vi "NI PXIe-411x PS Ch Page.vi"(8 "error in (no error)":errorcluster, 11 "Node Ptr":T2 format="%.0x") -> (0 "error out":errorcluster)   [LabVIEW 2023, in "NI PXIe-411x PS Custom Device.lvlib"]
uses:
  NI PXIe-411x PS Custom Device.lvlib
  <vilib>/NI VeriStand/Custom Device API/Custom Device Item Ref.ctl
  411x_Channel #.ctl
  411x_Global.vi
  <vilib>/NI VeriStand/Custom Device API/Get Item Property (Boolean).vi
  <vilib>/NI VeriStand/Custom Device API/Get Item Property (U16).vi
  <vilib>/NI VeriStand/Custom Device API/Get Item Property (Double).vi
  <vilib>/NI VeriStand/Custom Device API/Get Item Property (I32).vi
  <vilib>/NI VeriStand/Custom Device API/Set Item Property (I32).vi
  <vilib>/NI VeriStand/Custom Device API/Set Item Property (U16).vi
  <vilib>/NI VeriStand/Custom Device API/Set Item Property (Double).vi
  <vilib>/NI VeriStand/Custom Device API/Custom Device API.lvlib
panel:
  in  "Sense":i32(ring) items=["Local"=1008, "Remote"=1009]
  in  "Channel #":T1
  in  "Voltage Limit":dbl caption="Range (0-6V)" format="%.4f"
  in  "Initial Current Value":dbl caption="Range (0.01 -1A)" format="%.4f"
  in  "Current Limit":dbl caption="Range (0.01-1A)" format="%.4f"
  in  "IO Type":enum16{"Voltage Output", "Current Output"}(ring)
  in  "Voltage Level":dbl caption="Range (0-6V)" format="%_4f"
  in  "Name":string
  in  "Header":cluster{"Section Name":string}={"Section Name"="PXI-4112  Settings"}
  in  "Description":string
  in  "Delete":bool
  # "Voltage  IO Settings"
  # "Current IO Settings"
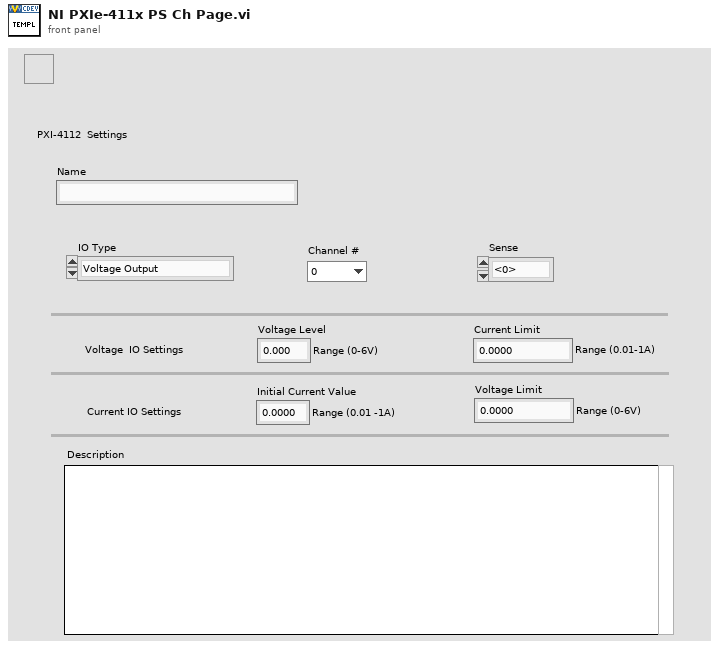
[diagram p1: front panel]
types:
  T1 = typedef "NI PXIe-411x PS Custom Device.lvlib/411x_Channel #.ctl" = enum16{"0", "1"}
  T2 = typedef "Custom Device API.lvlib/Custom Device Item Ref.ctl" = u64
  T3 = enum8{"Enabled", "Disabled", "Disabled and Grayed Out"}
  T4 = cluster{"V_min":dbl, "V_max":dbl, "I_min":dbl, "I_max":dbl}
  T5 = typedef "Custom Device API.lvlib/Custom Device Item Info.ctl" = cluster{"Name":string, "Is Channel":bool, "GUID":string, "Is Waveform":bool}
  T6 = typedef "Custom Device API.lvlib/Custom Device Commands.ctl" = enum16{"Default", "Item renamed", "Shutdown", "Dynamic button pressed"}
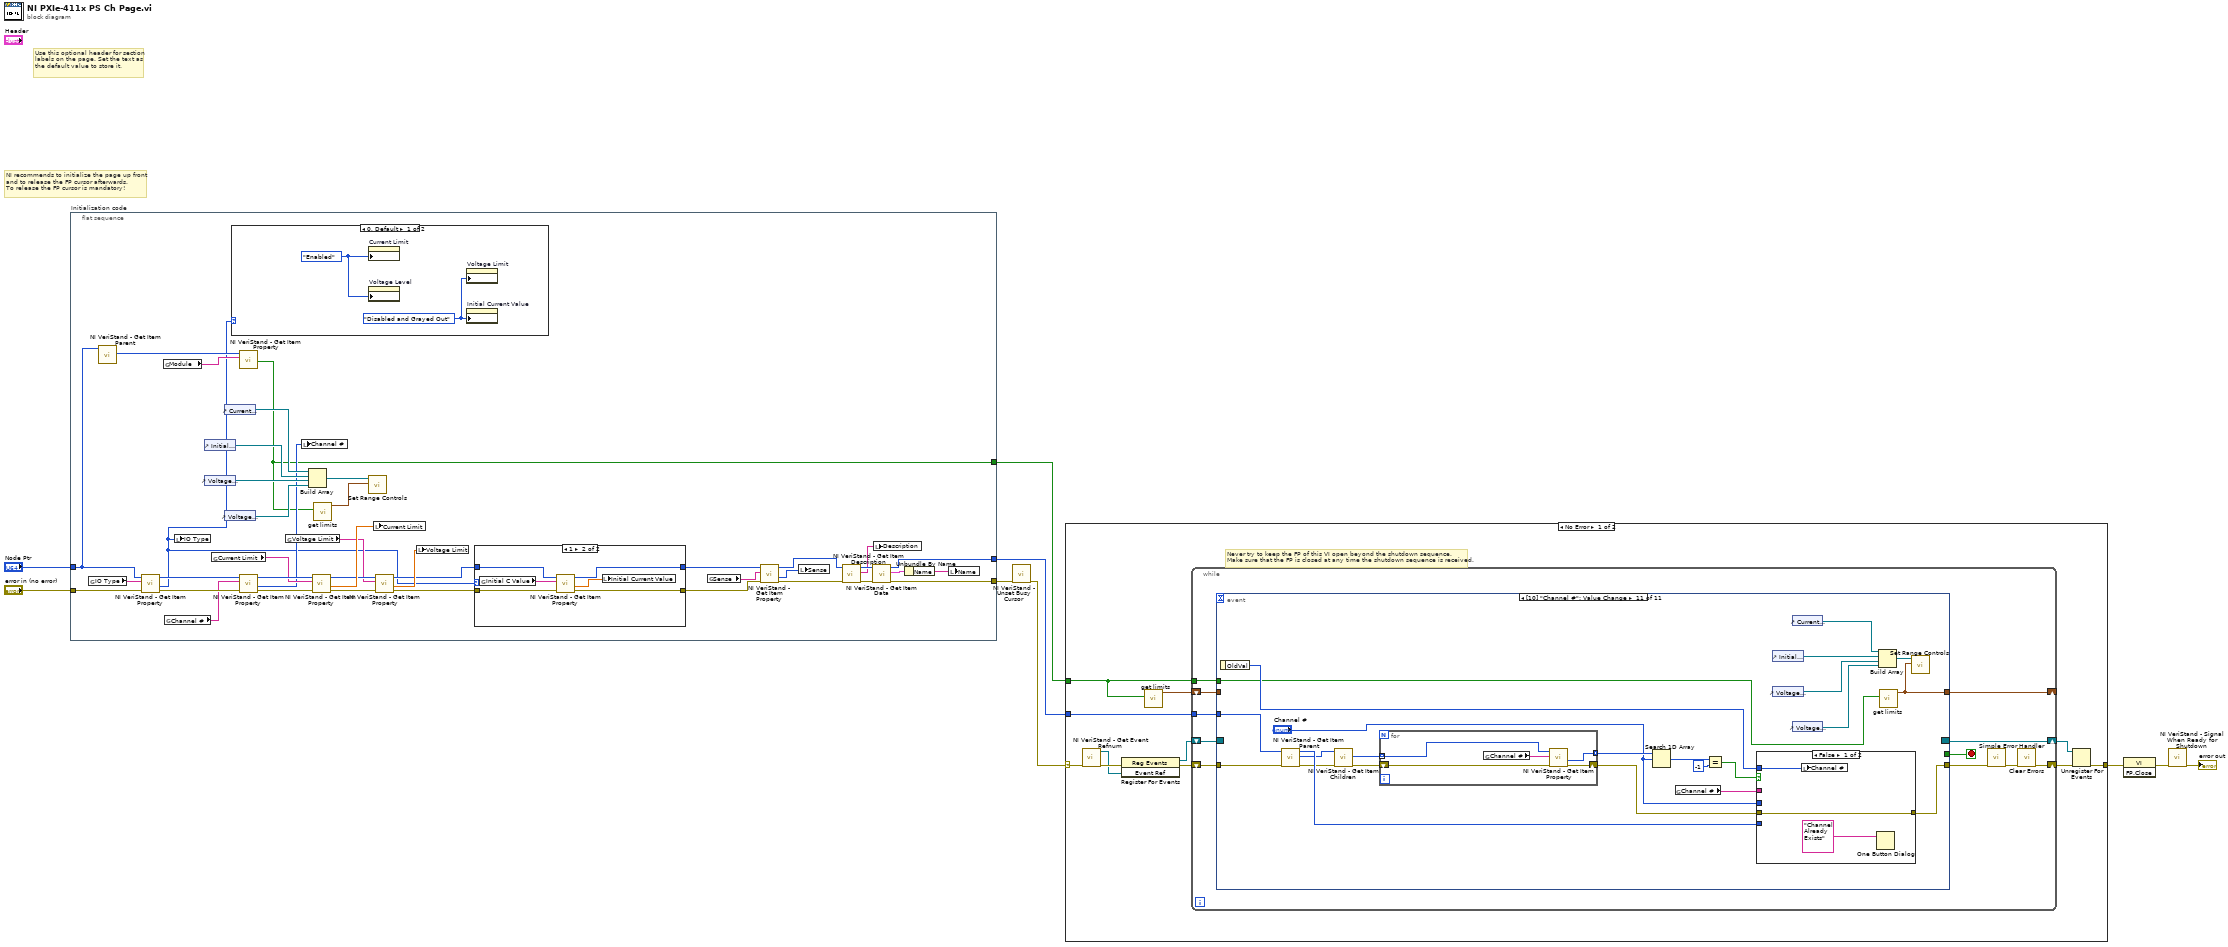
[diagram p0: block diagram]
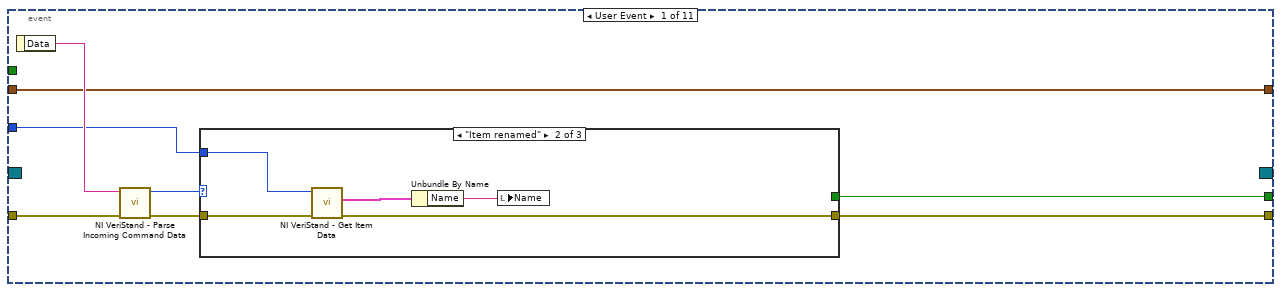
[diagram p2: hidden frame]
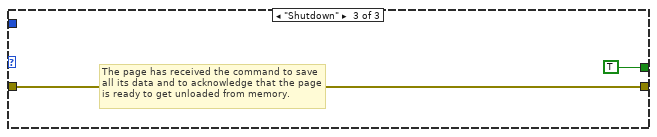
[diagram p4: hidden frame]
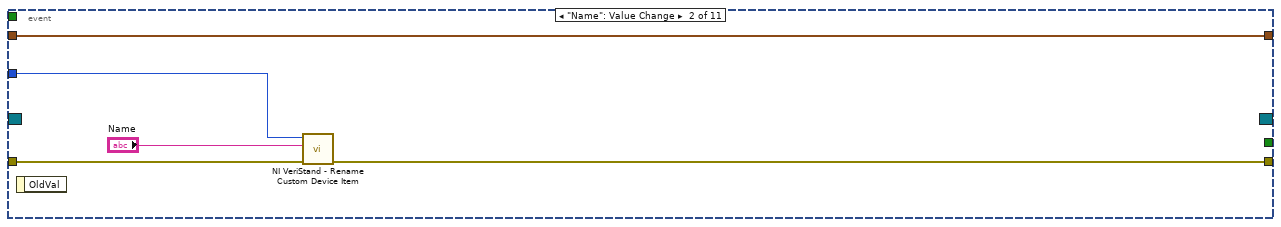
[diagram p5: hidden frame]
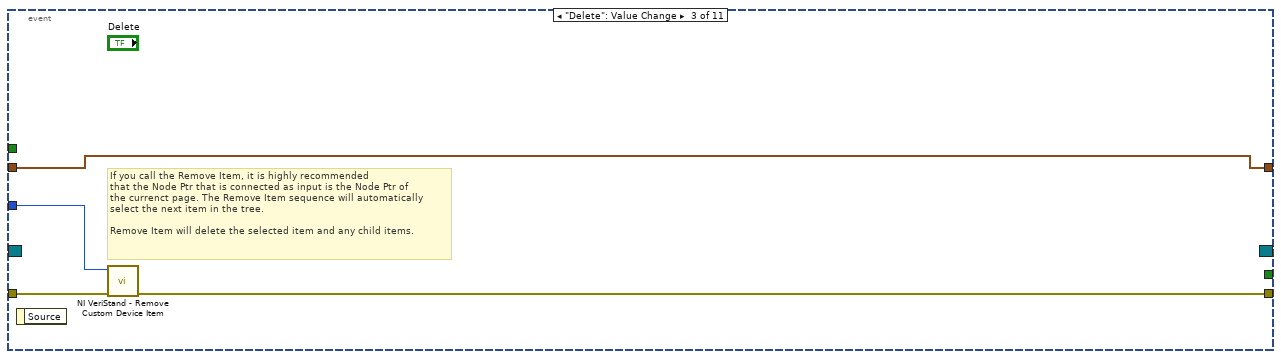
[diagram p6: hidden frame]
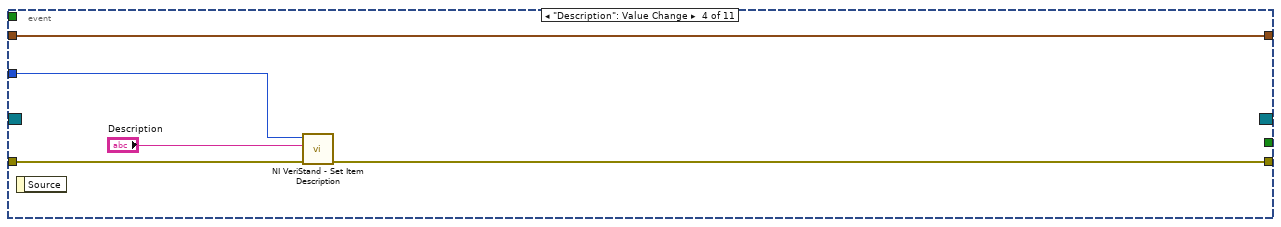
[diagram p7: hidden frame]
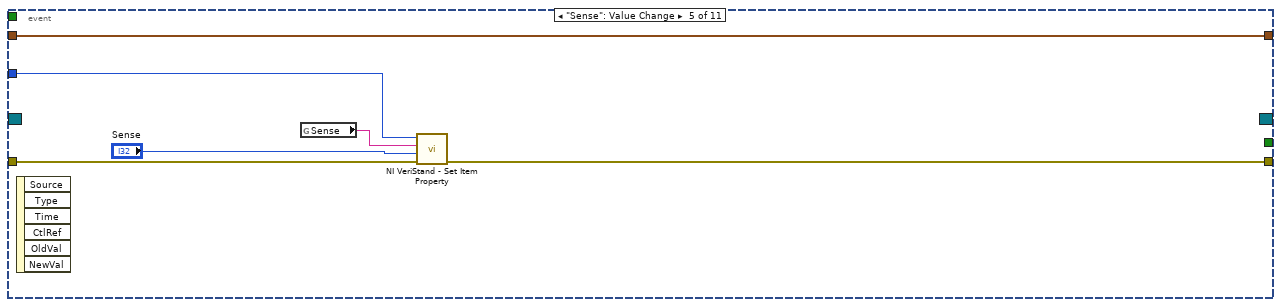
[diagram p8: hidden frame]
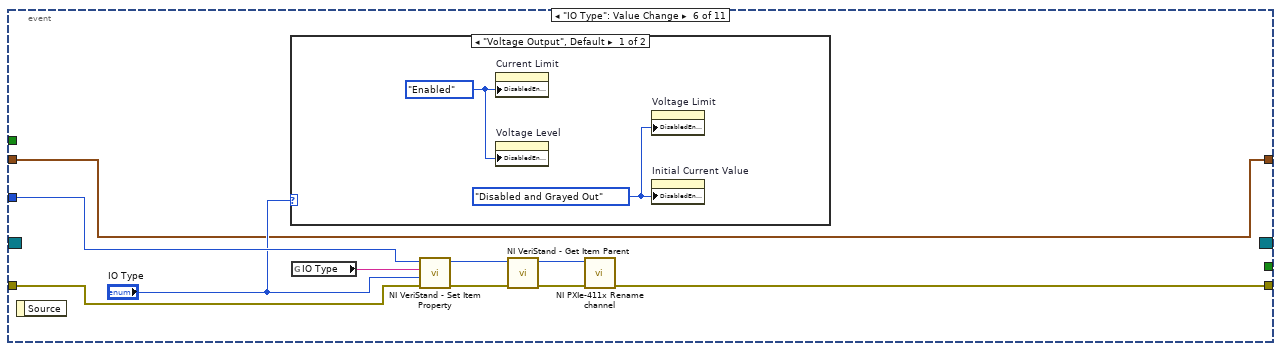
[diagram p9: hidden frame]
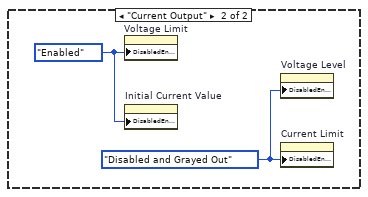
[diagram p10: hidden frame]
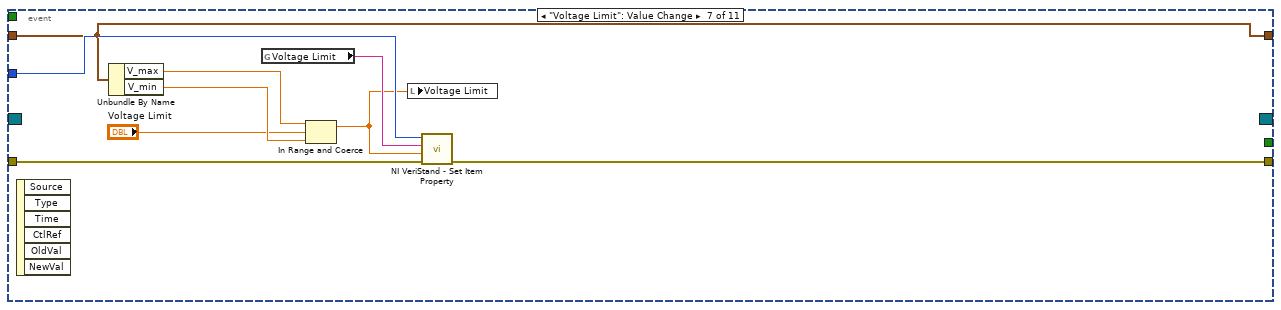
[diagram p11: hidden frame]
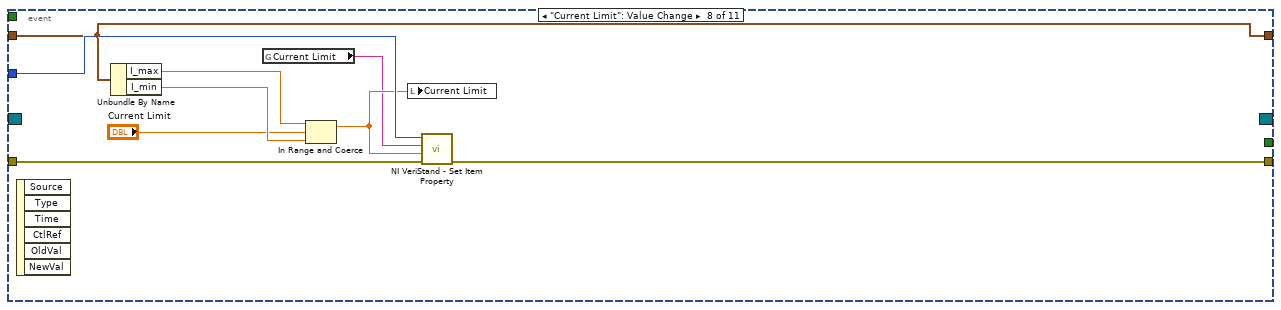
[diagram p12: hidden frame]
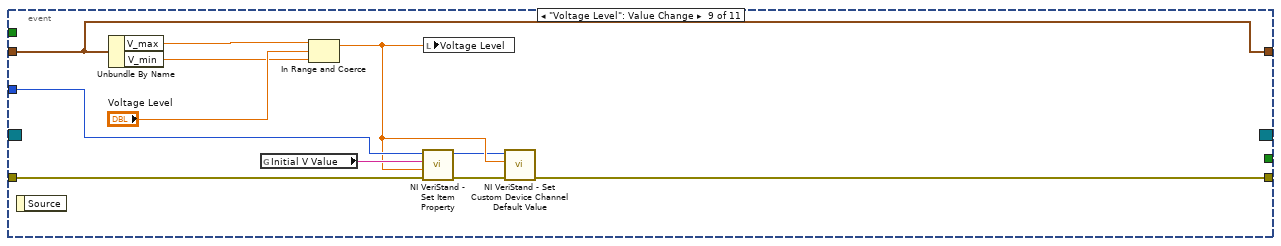
[diagram p13: hidden frame]
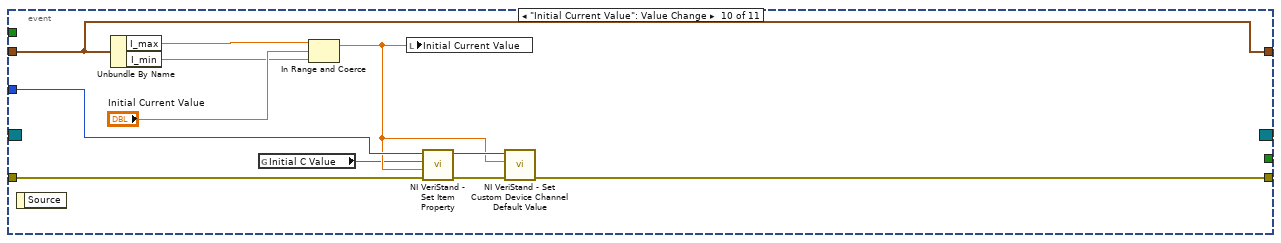
[diagram p14: hidden frame]
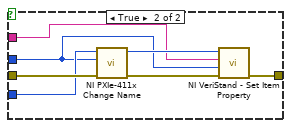
[diagram p15: hidden frame]
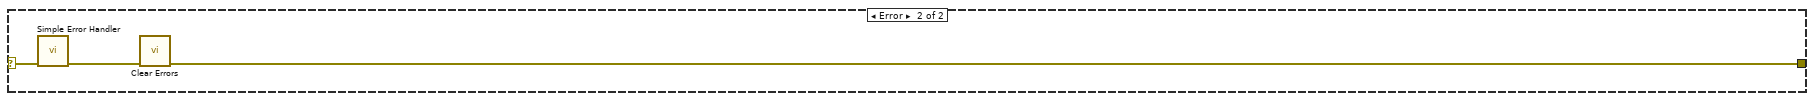
[diagram p16: hidden frame]
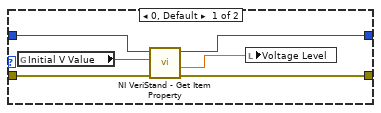
[diagram p17: hidden frame]
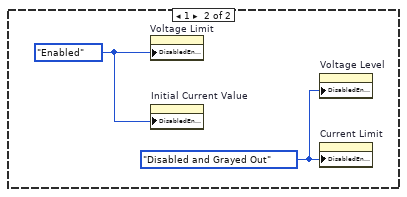
[diagram p18: hidden frame]
diagram:
  # "Use this optional header for section labels on the page. Set the text as the default value to store it."
  # "NI recommends to initialize the page up front\nand to release the FP cursor afterwards.\nTo release the FP cursor is mandatory!"
  n1 = flat-sequence "Initialization code" {
    tunnel: "error in (no error)" -> [w42]
    tunnel: "Node Ptr" -> [w21]
    tunnel: [w44] -> w5
    tunnel: [w49] -> w3
    tunnel: [w11] -> w1
    frame #0 {
      n2 = global read "411x_Global.vi" "IO Type"() -> (w41:string)
      n3 = call <vilib>:"NI VeriStand - Get Item Parent.vi"("Item Ref in"=w21) -> ("Parent Ref"=w19:T2)  [unwired: 7 in, 3 out]
      n4 = call-poly <vilib>:"NI VeriStand - Get Item Property.vi"("error in (no error)"=w42, "Property Name"=w41, "Item Ref in"=w21) -> ("error out"=w40:errorcluster, "Value"=w10:u16, "Item Ref out"=w39:T2)  [unwired: 5 in, 1 out]
      n5 = global read "411x_Global.vi" "Module"() -> (w20:string)
      n6 = global read "411x_Global.vi" "Channel #"() -> (w38:string)
      n7 = local write "IO Type"(w10) -> ()
      n8 = control-ref of="Initial Current Value"() -> (w15:refnum<vi>)
      n9 = control-ref of="Voltage Level"() -> (w16:refnum<vi>)
      n10 = global read "411x_Global.vi" "Current Limit"() -> (w35:string)
      n11 = control-ref of="Current Limit"() -> (w14:refnum<vi>)
      n12 = control-ref of="Voltage Limit"() -> (w17:refnum<vi>)
      n13 = case shown="0, Default" w10 {
        frame 0, Default {
          w62 = T3."Enabled" ("Disabled")
          w63 = T3."Disabled and Grayed Out" ("Disabled")
          n14 = property on="Current Limit" class="DigNum (strict)"("DisabledEnum"=w62) -> ()  [unwired: 2 in, 2 out]
          n15 = property on="Voltage Level" class="DigNum (strict)"("DisabledEnum"=w62) -> ()  [unwired: 2 in, 2 out]
          n16 = property on="Voltage Limit" class="DigNum (strict)"("DisabledEnum"=w63) -> ()  [unwired: 2 in, 2 out]
          n17 = property on="Initial Current Value" class="DigNum (strict)"("DisabledEnum"=w63) -> ()  [unwired: 2 in, 2 out]
        }
        frame 1 {
          w64 = T3."Enabled" ("Disabled")
          w65 = T3."Disabled and Grayed Out" ("Disabled")
          n18 = property on="Voltage Limit" class="DigNum (strict)"("DisabledEnum"=w64) -> ()  [unwired: 2 in, 2 out]
          n19 = property on="Initial Current Value" class="DigNum (strict)"("DisabledEnum"=w64) -> ()  [unwired: 2 in, 2 out]
          n20 = property on="Voltage Level" class="DigNum (strict)"("DisabledEnum"=w65) -> ()  [unwired: 2 in, 2 out]
          n21 = property on="Current Limit" class="DigNum (strict)"("DisabledEnum"=w65) -> ()  [unwired: 2 in, 2 out]
        }
      }
      n22 = call-poly <vilib>:"NI VeriStand - Get Item Property.vi"("Property Name"=w20, "Item Ref in"=w19) -> ("Value"=w11:bool)  [unwired: 6 in, 3 out]
      n23 = call-poly <vilib>:"NI VeriStand - Get Item Property.vi"("error in (no error)"=w40, "Property Name"=w38, "Item Ref in"=w39) -> ("error out"=w36:errorcluster, "Value"=w12:u16, "Item Ref out"=w37:T2)  [unwired: 5 in, 1 out]
      n24 = global read "411x_Global.vi" "Voltage Limit"() -> (w31:string)
      n25 = local write "Channel #"(w12) -> ()
      n26 = Build Array(w14, w15, w16, w17) -> (w18:refnum<vi>[])
      n27 = call-poly <vilib>:"NI VeriStand - Get Item Property.vi"("error in (no error)"=w36, "Property Name"=w35, "Item Ref in"=w37) -> ("error out"=w33:errorcluster, "Value"=w34:dbl, "Item Ref out"=w32:T2)  [unwired: 5 in, 1 out]
      n28 = call "get limits.vi"("4112?"=w11) -> ("output cluster"=w13:T4)  [unwired: 10 in]
      n29 = call "Set Range Controls.vi"("Ranges"=w13, "Reference Array"=w18) -> ()  [unwired: 10 in]
      n30 = local write "Current Limit"(w34) -> ()
      n31 = call-poly <vilib>:"NI VeriStand - Get Item Property.vi"("error in (no error)"=w33, "Property Name"=w31, "Item Ref in"=w32) -> ("error out"=w28:errorcluster, "Value"=w30:dbl, "Item Ref out"=w29:T2)  [unwired: 5 in, 1 out]
      n32 = local write "Voltage Limit"(w30) -> ()
      n33 = case shown="1" w10 {
        tunnel: w29 -> [w55 w61]
        tunnel: w28 -> [w54 w60]
        tunnel: [w53 w59] -> w26
        tunnel: [w52 w58] -> w25
        frame 0, Default {
          n34 = global read "411x_Global.vi" "Initial V Value"() -> (w51:string)
          n35 = call-poly <vilib>:"NI VeriStand - Get Item Property.vi"("error in (no error)"=w54, "Property Name"=w51, "Item Ref in"=w55) -> ("error out"=w53:errorcluster, "Value"=w50:dbl, "Item Ref out"=w52:T2)  [unwired: 5 in, 1 out]
          n36 = local write "Voltage Level"(w50) -> ()
        }
        frame 1 {
          n37 = global read "411x_Global.vi" "Initial C Value"() -> (w57:string)
          n38 = call-poly <vilib>:"NI VeriStand - Get Item Property.vi"("error in (no error)"=w60, "Property Name"=w57, "Item Ref in"=w61) -> ("error out"=w59:errorcluster, "Value"=w56:dbl, "Item Ref out"=w58:T2)  [unwired: 5 in, 1 out]
          n39 = local write "Initial Current Value"(w56) -> ()
        }
      }
      n40 = global read "411x_Global.vi" "Sense"() -> (w24:string)
      n41 = call-poly <vilib>:"NI VeriStand - Get Item Property.vi"("error in (no error)"=w26, "Property Name"=w24, "Item Ref in"=w25) -> ("error out"=w22:errorcluster, "Value"=w27:i32, "Item Ref out"=w23:T2)  [unwired: 5 in, 1 out]
      n42 = local write "Sense"(w27) -> ()
      n43 = call <vilib>:"NI VeriStand - Get Item Description.vi"("error in (no error)"=w22, "Item Ref in"=w23) -> ("error out"=w46:errorcluster, "Description"=w47:string, "Item Ref out"=w48:T2)  [unwired: 7 out]
      n44 = call <vilib>:"NI VeriStand - Get Item Data.vi"("error in (no error)"=w46, "Item Ref in"=w48) -> ("error out"=w44:errorcluster, "Item Info"=w45:T5, "Item Ref out"=w49:T2)  [unwired: 7 out]
      n45 = local write "Description"(w47) -> ()
      n46 = Unbundle By Name(w45) -> ("Name"=w43:string)
      n47 = local write "Name"(w43) -> ()
    }
  }
  n48 = call <vilib>:"NI VeriStand - Unset Busy Cursor.vi"("error in (no error)"=w5) -> ("error out"=w4:errorcluster)  [unwired: 10 out]
  n49 = case shown="No Error" w4 {
    selector: w4 -> [w68 w218]
    tunnel: [w73 w216] -> w9
    tunnel: w3 -> [w69 _]
    tunnel: w1 -> [w66 _]
    frame No Error {
      # "Never try to keep the FP of this VI open beyond the shutdown sequence.\nMake sure that the FP is closed at any time the shutdown sequence is received."
      n50 = call <vilib>:"NI VeriStand - Get Event Refnum.vi"("error in (no error)"=w68) -> ("error out"=w76:errorcluster, "Event Ref"=w72:refnum<user-event>)  [unwired: 9 out]
      n51 = register-events(error in=w76, w72) -> (reference out=w70:refnum<event-registration>, error out=w71:errorcluster)  [unwired: 1 in]
      n52 = call "get limits.vi"("4112?"=w66) -> ("output cluster"=w67:T4)  [unwired: 10 in]
      n53 = while {
        tunnel: w69 -> [w83]
        shift-right: [w80] -> w74
        shift-left: w71 -> [w86]
        shift-right: [w87] -> w75
        shift-left: w70 -> [w85]
        shift-right: [w79] -> _
        shift-left: w67 -> [w78]
        tunnel: w66 -> [w77]
        stop <- w84 stop-if-true
        n54 = event shown="[10] \"Channel #\": Value Change" {
          selector: w85 -> [_ _ _ _ _ _ _ _ _ _ _]
          dyn-events: [_ _ _ _ _ _ _ _ _ _ _] -> w87
          timeout: _ -> [_ _ _ _ _ _ _ _ _ _ _]
          tunnel: w86 -> [w95 w108 w112 w116 w123 w132 w145 w154 w165 w176 w187]
          tunnel: [w91 _ _ _ _ _ _ _ _ _ _] -> w84
          tunnel: [w90 w107 w111 w115 w122 w126 w144 w153 w162 w174 w186] -> w82
          tunnel: w83 -> [w89 w106 w110 w117 w121 w133 w146 w155 w166 w177 w188]
          tunnel: [w88 w104 w109 w113 w120 w124 w142 w150 w158 w171 w178] -> w79
          tunnel: w78 -> [w88 w104 w109 w113 w120 w124 w142 w150 w158 w171 _]
          tunnel: w77 -> [_ _ _ _ _ _ _ _ _ _ w184]
          event User Event {
            n55 = event-data() -> ("Data"=w94:string)  [unwired: 1 out]
            n56 = call <vilib>:"NI VeriStand - Parse Incoming Command Data.vi"("error in (no error)"=w95, "Incoming data"=w94) -> ("error out"=w93:errorcluster, "Action"=w92:T6)  [unwired: 8 out]
            n57 = case shown="\"Item renamed\"" w92 {
              tunnel: w93 -> [w96 w101 w102]
              tunnel: [_ _ TRUE] -> w91
              tunnel: [w96 w98 w102] -> w90
              tunnel: w89 -> [_ w100 _]
              frame "Default", Default {
              }
              frame "Item renamed" {
                n58 = call <vilib>:"NI VeriStand - Get Item Data.vi"("error in (no error)"=w101, "Item Ref in"=w100) -> ("error out"=w98:errorcluster, "Item Info"=w99:T5)  [unwired: 8 out]
                n59 = Unbundle By Name(w99) -> ("Name"=w97:string)
                n60 = local write "Name"(w97) -> ()
              }
              frame "Shutdown" {
                # "The page has received the command to save all its data and to acknowledge that the page is ready to get unloaded from memory."
              }
            }
          }
          event "Name": Value Change {
            n61 = event-data() -> ()  [unwired: 2 out]
            n62 = call <vilib>:"NI VeriStand - Rename Custom Device Item.vi"("error in (no error)"=w108, "New Name"="Name", "Item Ref in"=w106) -> ("error out"=w107:errorcluster)  [unwired: 1 in, 7 out]
          }
          event "Delete": Value Change {
            # "If you call the Remove Item, it is highly recommended\nthat the Node Ptr that is connected as input is the Node Ptr of\nthe currenct page. The Remove Item sequence will automatically\nselect the next item in the tree.\n\nRemove Item will delete the selected item and any child items."
            n63 = event-data() -> ()  [unwired: 2 out]
            n64 = call <vilib>:"NI VeriStand - Remove Custom Device Item.vi"("error in (no error)"=w112, "Item Ref in"=w110) -> ("error out"=w111:errorcluster)  [unwired: 1 in, 8 out]
          }
          event "Description": Value Change {
            n65 = event-data() -> ()  [unwired: 2 out]
            n66 = call <vilib>:"NI VeriStand - Set Item Description.vi"("error in (no error)"=w116, "Description"="Description", "Item Ref in"=w117) -> ("error out"=w115:errorcluster)  [unwired: 8 out]
          }
          event "Sense": Value Change {
            n67 = event-data() -> ()  [unwired: 7 out]
            n68 = global read "411x_Global.vi" "Sense"() -> (w119:string)
            n69 = call-poly <vilib>:"NI VeriStand - Set Item Property.vi"("error in (no error)"=w123, "Value"="Sense", "Property Name"=w119, "Item Ref in"=w121) -> ("error out"=w122:errorcluster)  [unwired: 5 in, 2 out]
          }
          event "IO Type": Value Change {
            n70 = event-data() -> ()  [unwired: 2 out]
            n71 = case shown="\"Voltage Output\", Default" "IO Type" {
              frame "Voltage Output", Default {
                w134 = T3."Enabled" ("Disabled")
                w135 = T3."Disabled and Grayed Out" ("Disabled")
                n72 = property on="Current Limit" class="DigNum (strict)"("DisabledEnum"=w134) -> ()  [unwired: 2 in, 2 out]
                n73 = property on="Voltage Level" class="DigNum (strict)"("DisabledEnum"=w134) -> ()  [unwired: 2 in, 2 out]
                n74 = property on="Voltage Limit" class="DigNum (strict)"("DisabledEnum"=w135) -> ()  [unwired: 2 in, 2 out]
                n75 = property on="Initial Current Value" class="DigNum (strict)"("DisabledEnum"=w135) -> ()  [unwired: 2 in, 2 out]
              }
              frame "Current Output" {
                w136 = T3."Enabled" ("Disabled")
                w137 = T3."Disabled and Grayed Out" ("Disabled")
                n76 = property on="Voltage Limit" class="DigNum (strict)"("DisabledEnum"=w136) -> ()  [unwired: 2 in, 2 out]
                n77 = property on="Initial Current Value" class="DigNum (strict)"("DisabledEnum"=w136) -> ()  [unwired: 2 in, 2 out]
                n78 = property on="Voltage Level" class="DigNum (strict)"("DisabledEnum"=w137) -> ()  [unwired: 2 in, 2 out]
                n79 = property on="Current Limit" class="DigNum (strict)"("DisabledEnum"=w137) -> ()  [unwired: 2 in, 2 out]
              }
            }
            n80 = global read "411x_Global.vi" "IO Type"() -> (w131:string)
            n81 = call-poly <vilib>:"NI VeriStand - Set Item Property.vi"("error in (no error)"=w132, "Value"="IO Type", "Property Name"=w131, "Item Ref in"=w133) -> ("error out"=w129:errorcluster, "Item Ref out"=w127:T2)  [unwired: 5 in, 1 out]
            n82 = call <vilib>:"NI VeriStand - Get Item Parent.vi"("error in (no error)"=w129, "Item Ref in"=w127) -> ("error out"=w125:errorcluster, "Item Ref out"=w128:T2)  [unwired: 6 in, 2 out]
            n83 = call "NI PXIe-411x Rename channel.vi"("error in (no error)"=w125, "Node Ptr"=w128) -> ("error out"=w126:errorcluster)  [unwired: 8 in, 1 out]
          }
          event "Voltage Limit": Value Change {
            n84 = event-data() -> ()  [unwired: 7 out]
            n85 = Unbundle By Name(w142) -> ("V_max"=w141:dbl, "V_min"=w140:dbl)
            n86 = global read "411x_Global.vi" "Voltage Limit"() -> (w143:string)
            n87 = In Range and Coerce(upper limit=w141, x="Voltage Limit", lower limit=w140) -> (coerced(x)=w138:dbl)  [unwired: 1 out]
            n88 = local write "Voltage Limit"(w138) -> ()
            n89 = call-poly <vilib>:"NI VeriStand - Set Item Property.vi"("error in (no error)"=w145, "Value"=w138, "Property Name"=w143, "Item Ref in"=w146) -> ("error out"=w144:errorcluster)  [unwired: 5 in, 2 out]
          }
          event "Current Limit": Value Change {
            n90 = event-data() -> ()  [unwired: 7 out]
            n91 = Unbundle By Name(w150) -> ("I_max"=w152:dbl, "I_min"=w151:dbl)
            n92 = global read "411x_Global.vi" "Current Limit"() -> (w147:string)
            n93 = In Range and Coerce(upper limit=w152, x="Current Limit", lower limit=w151) -> (coerced(x)=w148:dbl)  [unwired: 1 out]
            n94 = local write "Current Limit"(w148) -> ()
            n95 = call-poly <vilib>:"NI VeriStand - Set Item Property.vi"("error in (no error)"=w154, "Value"=w148, "Property Name"=w147, "Item Ref in"=w155) -> ("error out"=w153:errorcluster)  [unwired: 5 in, 2 out]
          }
          event "Voltage Level": Value Change {
            n96 = event-data() -> ()  [unwired: 2 out]
            n97 = Unbundle By Name(w158) -> ("V_max"=w157:dbl, "V_min"=w156:dbl)
            n98 = global read "411x_Global.vi" "Initial V Value"() -> (w164:string)
            n99 = In Range and Coerce(upper limit=w157, x="Voltage Level", lower limit=w156) -> (coerced(x)=w161:dbl)  [unwired: 1 out]
            n100 = call-poly <vilib>:"NI VeriStand - Set Item Property.vi"("error in (no error)"=w165, "Value"=w161, "Property Name"=w164, "Item Ref in"=w166) -> ("error out"=w163:errorcluster, "Item Ref out"=w160:T2)  [unwired: 5 in, 1 out]
            n101 = local write "Voltage Level"(w161) -> ()
            n102 = call <vilib>:"NI VeriStand - Set Custom Device Channel Default Value.vi"("error in (no error)"=w163, "Default Value"=w161, "Channel Ref in"=w160) -> ("error out"=w162:errorcluster)  [unwired: 7 in, 1 out]
          }
          event "Initial Current Value": Value Change {
            n103 = event-data() -> ()  [unwired: 2 out]
            n104 = Unbundle By Name(w171) -> ("I_max"=w170:dbl, "I_min"=w169:dbl)
            n105 = global read "411x_Global.vi" "Initial C Value"() -> (w167:string)
            n106 = In Range and Coerce(upper limit=w170, x="Initial Current Value", lower limit=w169) -> (coerced(x)=w168:dbl)  [unwired: 1 out]
            n107 = local write "Initial Current Value"(w168) -> ()
            n108 = call-poly <vilib>:"NI VeriStand - Set Item Property.vi"("error in (no error)"=w176, "Value"=w168, "Property Name"=w167, "Item Ref in"=w177) -> ("error out"=w175:errorcluster, "Item Ref out"=w173:T2)  [unwired: 5 in, 1 out]
            n109 = call <vilib>:"NI VeriStand - Set Custom Device Channel Default Value.vi"("error in (no error)"=w175, "Default Value"=w168, "Channel Ref in"=w173) -> ("error out"=w174:errorcluster)  [unwired: 7 in, 1 out]
          }
          event Value Change {
            n110 = event-data() -> ("OldVal"=w190:T1)  [unwired: 1 out]
            n111 = call <vilib>:"NI VeriStand - Get Item Parent.vi"("error in (no error)"=w187, "Item Ref in"=w188) -> ("error out"=w191:errorcluster, "Parent Ref"=w192:T2, "Item Ref out"=w200:T2)  [unwired: 6 in, 1 out]
            n112 = call <vilib>:"NI VeriStand - Get Item Children.vi"("error in (no error)"=w191, "Item Ref in"=w192) -> ("error out"=w194:errorcluster, "Child Refs"=w193:T2[])  [unwired: 6 in, 2 out]
            n113 = for {
              tunnel: w193 -> [w213] mode=indexing
              shift-right: [w214] -> w199
              shift-left: w194 -> [w215]
              tunnel: [w212] -> w195 mode=indexing
              n114 = global read "411x_Global.vi" "Channel #"() -> (w211:string)
              n115 = call-poly <vilib>:"NI VeriStand - Get Item Property.vi"("error in (no error)"=w215, "Property Name"=w211, "Item Ref in"=w213) -> ("error out"=w214:errorcluster, "Value"=w212:u16)  [unwired: 5 in, 2 out]
            }
            n116 = Search 1D Array(1D array=w195, element="Channel #") -> (index of element=w196:i32)  [unwired: 1 in]
            n117 = global read "411x_Global.vi" "Channel #"() -> (w189:string)
            n118 = Equal?(x=w196, y=-1) -> (x = y?=w198:bool)
            n119 = case shown="False" w198 {
              tunnel: w199 -> [w202 w210]
              tunnel: w200 -> [_ w209]
              tunnel: w189 -> [_ w205]
              tunnel: "Channel #" -> [_ w204]
              tunnel: [w202 w207] -> w186
              tunnel: w190 -> [w203 _]
              frame False {
                n120 = local write "Channel #"(w203) -> ()
                n121 = One Button Dialog(message="Channel Already Exists") -> ()  [unwired: 1 in, 1 out]
              }
              frame True {
                n122 = call "NI PXIe-411x Change Name.vi"("error in (no error)"=w210, "New #"=w204, "Node Ptr"=w209) -> ("error out"=w208:errorcluster, "Node Ptr out"=w206:T2)  [unwired: 7 in]
                n123 = call-poly <vilib>:"NI VeriStand - Set Item Property.vi"("error in (no error)"=w208, "Value"=w204, "Property Name"=w205, "Item Ref in"=w206) -> ("error out"=w207:errorcluster)  [unwired: 5 in, 2 out]
              }
            }
            n124 = control-ref of="Initial Current Value"() -> (w182:refnum<vi>)
            n125 = control-ref of="Voltage Level"() -> (w181:refnum<vi>)
            n126 = control-ref of="Current Limit"() -> (w183:refnum<vi>)
            n127 = control-ref of="Voltage Limit"() -> (w180:refnum<vi>)
            n128 = Build Array(w183, w182, w181, w180) -> (w179:refnum<vi>[])
            n129 = call "get limits.vi"("4112?"=w184) -> ("output cluster"=w178:T4)  [unwired: 10 in]
            n130 = call "Set Range Controls.vi"("Ranges"=w178, "Reference Array"=w179) -> ()  [unwired: 10 in]
          }
        }
        n131 = call <vilib>:"Simple Error Handler.vi"("error in (no error)"=w82) -> ("error out"=w81:errorcluster)  [unwired: 1 in, 7 out]
        n132 = call <vilib>:"Clear Errors.vi"("error in (no error)"=w81) -> ("error out"=w80:errorcluster)  [unwired: 1 in, 5 out]
      }
      n133 = Unregister For Events(event registration refnum=w75, error in=w74) -> (error out=w73:errorcluster)
    }
    frame Error {
      n134 = call <vilib>:"Simple Error Handler.vi"("error in (no error)"=w218) -> ("error out"=w217:errorcluster)  [unwired: 1 in, 7 out]
      n135 = call <vilib>:"Clear Errors.vi"("error in (no error)"=w217) -> ("error out"=w216:errorcluster)  [unwired: 1 in, 5 out]
    }
  }
  n136 = invoke class="VI" method="FP.Close"(error in=w9) -> (error out=w8:errorcluster)  [unwired: 2 in, 2 out]
  n137 = call <vilib>:"NI VeriStand - Signal When Ready for Shutdown.vi"("error in (no error)"=w8) -> ("error out"=→"error out":errorcluster)  [unwired: 10 out]
